vi "GetAcquisitionStatus.vi"(8 "error in":errorcluster, 11 "connection ID in":refnum<k5>) -> (0 "error out":errorcluster, 1 "Error Info":T1, 2 "Number of Points":i32, 3 "connection ID out":refnum<k5>, 4 "Log String":string, 5 "Finished":bool)   [LabVIEW 2020, in "ProdigyRemoteControl.lvlib"]
uses:
  ProdigyRemoteControl.lvlib
  DEFINITIONS/DEF_RcError.ctl
  DEFINITIONS/DEF_RcCmd.ctl
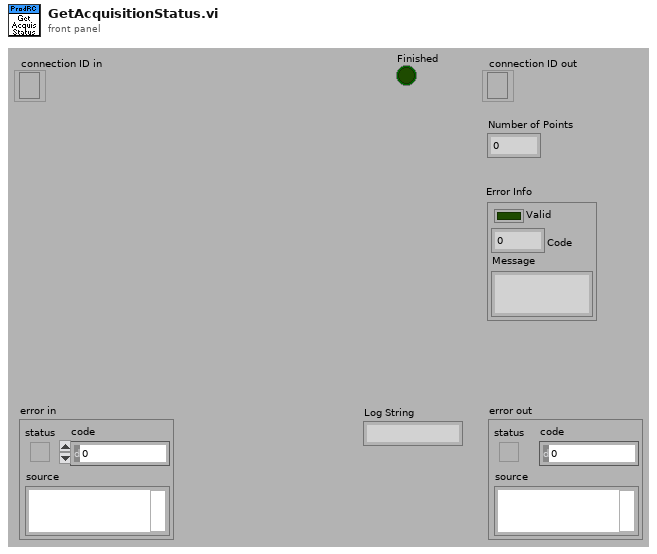
[diagram p1: front panel]
types:
  T1 = typedef "ProdigyRemoteControl.lvlib/DEF_RcError.ctl" = cluster{"Valid":bool, "Code":u16, "Message":string}
  T2 = typedef "ProdigyRemoteControl.lvlib/DEF_RcCmd.ctl" = string
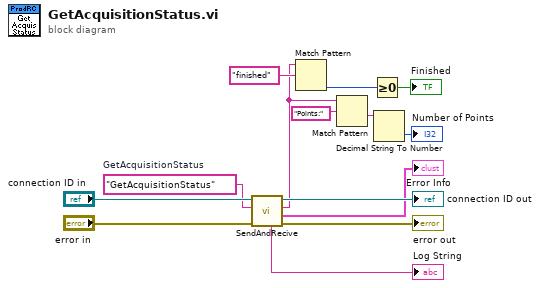
[diagram p0: block diagram]
diagram:
  w10 = T2 "GetAcquisitionStatus"  # GetAcquisitionStatus
  n1 = call "SendAndRecive.vi"("error in"="error in", "Command"=w10, "connection ID in"="connection ID in") -> ("error out"=→"error out":errorcluster, "Error Info"=→"Error Info":T1, "Answer"=w1:string, "connection ID out"=→"connection ID out":refnum<k5>, "Log String"=→"Log String":string)  [unwired: 4 in]
  n2 = Match Pattern(string=w1, regular expression="finished") -> (offset past match=w6:i32)  [unwired: 1 in, 3 out]
  n3 = Match Pattern(string=w1, regular expression="Points:") -> (after substring=w3:string)  [unwired: 1 in, 3 out]
  n4 = Greater Or Equal To 0?(x=w6) -> (x >= 0?=→"Finished":bool)
  n5 = Decimal String To Number(string=w3) -> (number=→"Number of Points":i32)  [unwired: 2 in, 1 out]
